vi "PWM Set Duty Cycle N Chans.vi"(8 "Error In":errorcluster, 9 "Duty Cycles":dbl[](array[numeric]), 10 "PWM Channels":u8[](array[numeric]), 11 "LINX Resource":T1) -> (0 "Error Out":errorcluster, 3 "LINX Resource":T1)   [LabVIEW 2014, in "LMH-LINX.lvlib"]
doc: "Set the duty cycle of the specified PWM channels. \n\nA duty cycle of 0 coresponds to 0% on and a duty cycle of 1 coresponds to 100% on."
uses:
  <vilib>/MakerHub/LINX/LMH-LINX.lvlib
  <vilib>/MakerHub/LINX/Private/Type Defs/LINX Ref.ctl
  <vilib>/MakerHub/LINX/Private/Type Defs/Platform.ctl
  <vilib>/MakerHub/LINX/Private/Type Defs/Interface.ctl
  <vilib>/MakerHub/LINX/Private/Device/Type Defs/LINX Device Config.ctl
  <vilib>/MakerHub/LINX/Private/Device/Type Defs/TCP Config.ctl
  <vilib>/MakerHub/LINX/Private/Device/Type Defs/Channels.ctl
  <vilib>/MakerHub/LINX/Private/Type Defs/Peripheral.ctl
  <vilib>/MakerHub/LINX/Private/Utilties/Generate Error.vi
  <vilib>/MakerHub/LINX/Private/Device/Device.lvlib
  <vilib>/MakerHub/LINX/Private/Local IO/Local IO.lvlib
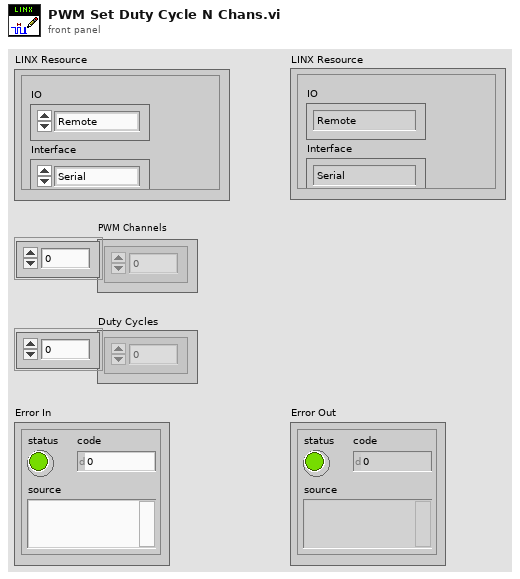
[diagram p1: front panel]
types:
  T1 = typedef "LMH-LINX.lvlib/LINX Ref.ctl" = cluster{"IO":T2, "Interface":T3, "LINX Device Config":T4}
  T2 = typedef "LMH-LINX.lvlib/Platform.ctl" = enum16{"Remote", "Local"}
  T3 = typedef "LMH-LINX.lvlib/Interface.ctl" = enum16{"Serial", "TCP"}
  T4 = typedef "LMH-LINX.lvlib/Device.lvlib/LINX Device Config.ctl" = cluster{"Interface":T3, "COM Port":refnum<visa-resource-name>, "TCP Configuration":T5, "Device Family":u8, "Device ID":u8, "Device Name":string, "TCP Ref":refnum<k5>, "Channels":T6}
  T5 = typedef "LMH-LINX.lvlib/Device.lvlib/TCP Config.ctl" = cluster{"IP Address":string, "Port":u16}
  T6 = typedef "LMH-LINX.lvlib/Channels.ctl" = cluster{"DI":u8[], "DO":u8[], "AI":u8[], "AO":u8[], "PWM":u8[], "QE":u8[], "UART":u8[], "I2C 2":u8[], "SPI":u8[], "CAN":u8[], "Servo":u8[], "AI Ref (V)":dbl, "AI Resolution (Bits)":u8, "AO Ref (V)":dbl, "AO Resolution (Bits)":u8}
  T7 = typedef "LMH-LINX.lvlib/Peripheral.ctl" = enum8{"DI", "DO", "AI", "AO", "PWM", "QE", "UART", "I2C", "SPI", "CAN", "Servo"}
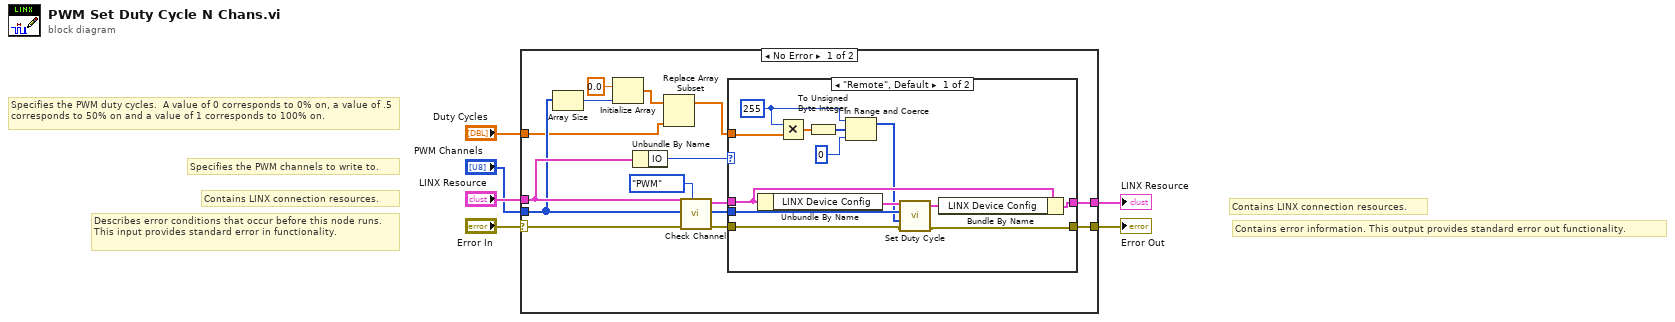
[diagram p0: block diagram]
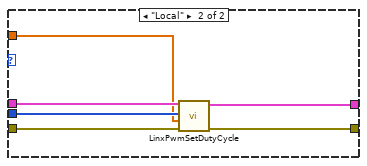
[diagram p2: hidden frame]
diagram:
  # "Specifies the PWM channels to write to."
  # "Specifies the PWM duty cycles.  A value of 0 corresponds to 0% on, a value of .5 corresponds to 50% on and a value of 1 corresponds to 100% on."
  # "Contains LINX connection resources."
  # "Contains error information. This output provides standard error out functionality."
  # "Contains LINX connection resources."
  # "Describes error conditions that occur before this node runs. This input provides standard error in functionality."
  n1 = case shown="No Error" "Error In" {
    selector: "Error In" -> [w13 w42]
    tunnel: [w20 w42] -> w6
    tunnel: [w19 w41] -> w5
    tunnel: "LINX Resource" -> [w17 w41]
    tunnel: "Duty Cycles" -> [w8 _]
    tunnel: "PWM Channels" -> [w12 _]
    frame No Error {
      n2 = Array Size(array=w12) -> (size(s)=w11:i32)
      n3 = Initialize Array(0.0 ("element"), w11) -> (w9:dbl[])
      n4 = Unbundle By Name(w17) -> ("IO"=w21:T2)
      n5 = Replace Array Subset(array=w9, new element=w8) -> (w7:dbl[])  [unwired: 1 in]
      n6 = call <vilib>:"Check Channel.vi"("Peripheral"=Peripheral."PWM", "Error In"=w13, "Channels"=w12, "LINX Resource"=w17) -> ("Error Out"=w15:errorcluster, "Channels"=w14:u8[], "LINX Resource"=w16:T1)  [unwired: 5 in]
      n7 = case shown="\"Remote\", Default" w21 {
        tunnel: w15 -> [w31 w37]
        tunnel: w16 -> [w34 w38]
        tunnel: [w32 w40] -> w20
        tunnel: [w33 w39] -> w19
        tunnel: w7 -> [w23 w35]
        tunnel: w14 -> [w28 w36]
        frame "Remote", Default {
          w24 = u8 255
          n8 = Unbundle By Name(w34) -> ("LINX Device Config"=w29:T4)
          n9 = Multiply(x=w24, y=w23) -> (x*y=w27:dbl[])
          n10 = To Unsigned Byte Integer(number=w27) -> (unsigned 8bit integer=w26:u8[])
          n11 = In Range and Coerce(upper limit=w24, x=w26, lower limit=u8 0) -> (coerced(x)=w22:u8[])  [unwired: 1 out]
          n12 = call <vilib>:"Set Duty Cycle.vi"("Error In"=w31, "Duty Cycles (0-255)"=w22, "Channels"=w28, "LINX Device Config"=w29) -> ("Error Out"=w32:errorcluster, "LINX Device Config"=w30:T4)  [unwired: 6 in]
          n13 = Bundle By Name(cluster=w34, "LINX Device Config"=w30) -> (w33:T1)
        }
        frame "Local" {
          n14 = call <vilib>:"LinxPwmSetDutyCycle.vi"("Error In"=w37, "Duty Cycles"=w35, "PWM Channels"=w36, "LINX Resource"=w38) -> ("Error Out"=w40:errorcluster, "LINX Resource"=w39:T1)  [unwired: 6 in]
        }
      }
    }
    frame Error {
    }
  }
  "Error Out" <- w6
  "LINX Resource" <- w5
